vi "ziExample-Module-AWG.vi"() -> ()   [LabVIEW 2009]
doc: "Control a Zurich instrument device via the LabOne Labview API. \nRequirements: Zurich Instruments UHFLI \nThis example shows how to start a AWG module and measure it with the scope module.\n\n© Zurich Instruments AG, www.zhinst.com"
uses:
  <instrlib>/Zurich Instruments LabOne/Public/Modules/ziTypeModEnum.ctl
  <instrlib>/Zurich Instruments LabOne/Public/Configure/ziSetValueDouble.vi
  <instrlib>/Zurich Instruments LabOne/Public/Configure/ziSetValueDoubleArray.vi
  <instrlib>/Zurich Instruments LabOne/Public/Modules/ziModSetValueBinary.vi
  <instrlib>/Zurich Instruments LabOne/Public/Modules/ziModSetValueDoubleArray.vi
  <instrlib>/Zurich Instruments LabOne/Public/Modules/ziModGetScopeWave.vi
  <instrlib>/Zurich Instruments LabOne/Zurich Instruments LabOne.lvlib
panel:
  out "Status":bool
  out "Finish":bool
  out "Scopeready":bool caption="scopeready"
  out "?":cluster{dbl[], "Data Float":sgl[]}[](graph)
  in  "AWG":string="// Define an integer constant\nconst N = 4096;\n// Create  Gaussian pulses with length N points,\n// amplitude +1.0, center at N/2, and a width of N/8\nwave gauss = 1.0*gauss(N, N/2, N/8);\n\nplayWave(gauss);\nsetTrigger(1);\nsetTrigger(0);"
  out "Error Out":errorcluster
  in  "Address":string="DEV"
  out "Selected Device":string
  # "ziExample-SweepModul.vi\nRequirements: UHFLI\nsee block diagram for VI description"
  # "Tested Devices:\n- UHFLI"
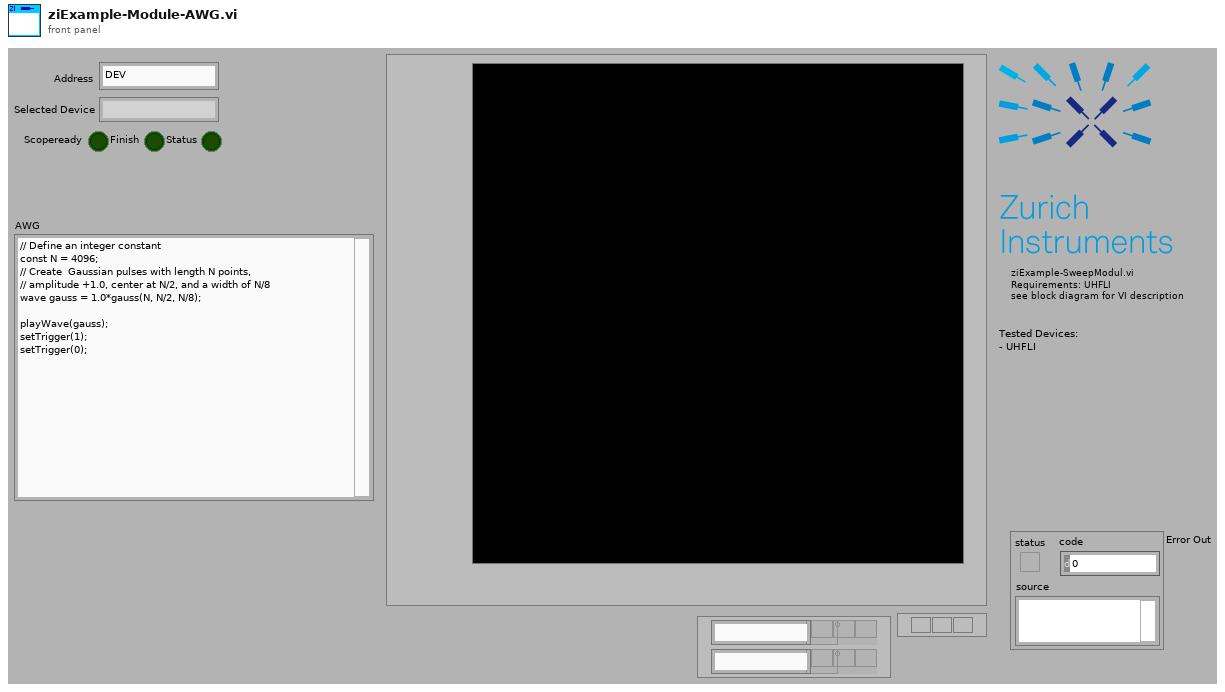
[diagram p1: front panel]
types:
  T1 = typedef "Zurich Instruments LabOne.lvlib/ziTypeModEnum.ctl" = u16
  T2 = typedef "Zurich Instruments LabOne.lvlib/ziTypeHandle.ctl" = cluster{"handleValid":bool, "Conn":u64, "Path Prefix":string, "Handle":u64, "Connected":bool, "Clockbase(s)":dbl}
  T3 = typedef "Zurich Instruments LabOne.lvlib/ziTypeModHandle.ctl" = cluster{"handleValid":bool, "Conn":u64, "ModHandle":u64, "moduleID":string, "Path Prefix":string}
  T4 = typedef "Zurich Instruments LabOne.lvlib/ziTypeModResults.ctl" = cluster{"PathArray":string[], "ValueType":T5, "NoOfResults":u64, "ziGenericHeader":T6[]}
  T5 = typedef "Zurich Instruments LabOne.lvlib/ziTypePollType.ctl" = enum16{"NONE", "DOUBLE_DATA", "INTEGER_DATA", "DEMOD_SAMPLE", "SCOPE_WAVE_HF2", "AUXIN_SAMPLE", "DIO_SAMPLE", "BYTE_ARRAY", "PWA_WAVE", "9", "10", "11", "12", "13", "14", "15", "TREE_CHANGE_DEPRI", "17", "ERROR", "19", "20", "21", "22", "23", "24", "25", "26", "27", "28", "29", "30", "31", "DOUBLE_DATA_TS", "INTEGER_DATA_TS", "34", "SCOPE_WAVE", "SCOPE_WAVE_EX", "37", "BYTE_ARRAY_TS", "39", "40", "41", "42", "43", "44", "45", "CNT_DATA", "47", "TREE_CHANGE", "49", "50", "51", "52", "53", "54", "55", "56", "57", "58", "59", "60", "61", "62", "63", "SWEEPER_DATA", "SPECTRUM_DATA", "ADVISOR_DATA", "VECTOR_DATA", "IMP_DATA"}
  T6 = typedef "Zurich Instruments LabOne.lvlib/ziTypeModGenericHeader.ctl" = cluster{"HeaderType":enum8{"HEADER_TYPE_NONE", "HEADER_TYPE_SWTRIGGER", "HEADER_TYPE_SWEEPER"}, "SampleFormat":u8, "SystemTime":timestamp, "CreatedTimeStamp":u64, "ChangedTimeStamp":u64, "Flags":u32, "ChunkSizeBytes":u64, "Name":string, "Status":u32, "GroupIndex":u32, "Color":u32, "ActiveRow":u32, "TriggerNumber":u64, "GridRows":u32, "GridCols":u32, "GridMode":u32, "GridOperation":u32, "GridDirection":u32, "GridRepetitions":u32, "GridColDelta":dbl, "GridColOffset":dbl, "GridRowDelta":dbl, "GridRowOffset":dbl, "Bandwidth":dbl, "Center":dbl, "Nenbw":dbl}
  T7 = typedef "Zurich Instruments LabOne.lvlib/ziTypeScopeWave.ctl" = cluster{"Timestamp (ticks)":u64, "Timestamp Trigger (ticks)":u64, "dt (s)":dbl, "Channel Enable":u8[], "Channel Input":enum8{"Signal Input 1", "Signal Input 2", "Trigger Input 1", "Trigger Input 2", "Aux Output 1", "Aux Output 2", "Aux Output 3", "Aux Output 4", "Aux Input 1", "Aux Input 2"}[], "Trigger Enable":u64, "Trigger Input":u64, "Channel BW Limit":u8[], "Channel Math":u8[], "Channel Scaling":sgl[], "Sequence Number":u32, "Segment Number":u32, "Block Number":u32, "Data Transfer Mode":enum8{"Single Transfer", "Block Transfer", "Continuous Transfer", "FFT Single Transfer"}, "Block Marker":enum8{"None", "End of Block"}, "Flags":u8, "Sample Format":enum8{"Int16", "Int32", "Float32", "reserved", "Int16 Interleaved", "Int32 Interleaved", "Float32 Interleaved"}, "Sample Count":u32, "Channel Offset":dbl[], "Data Int16":i16[], "Data Int32":i32[], "Data Float":sgl[], "Total Samples":u64}
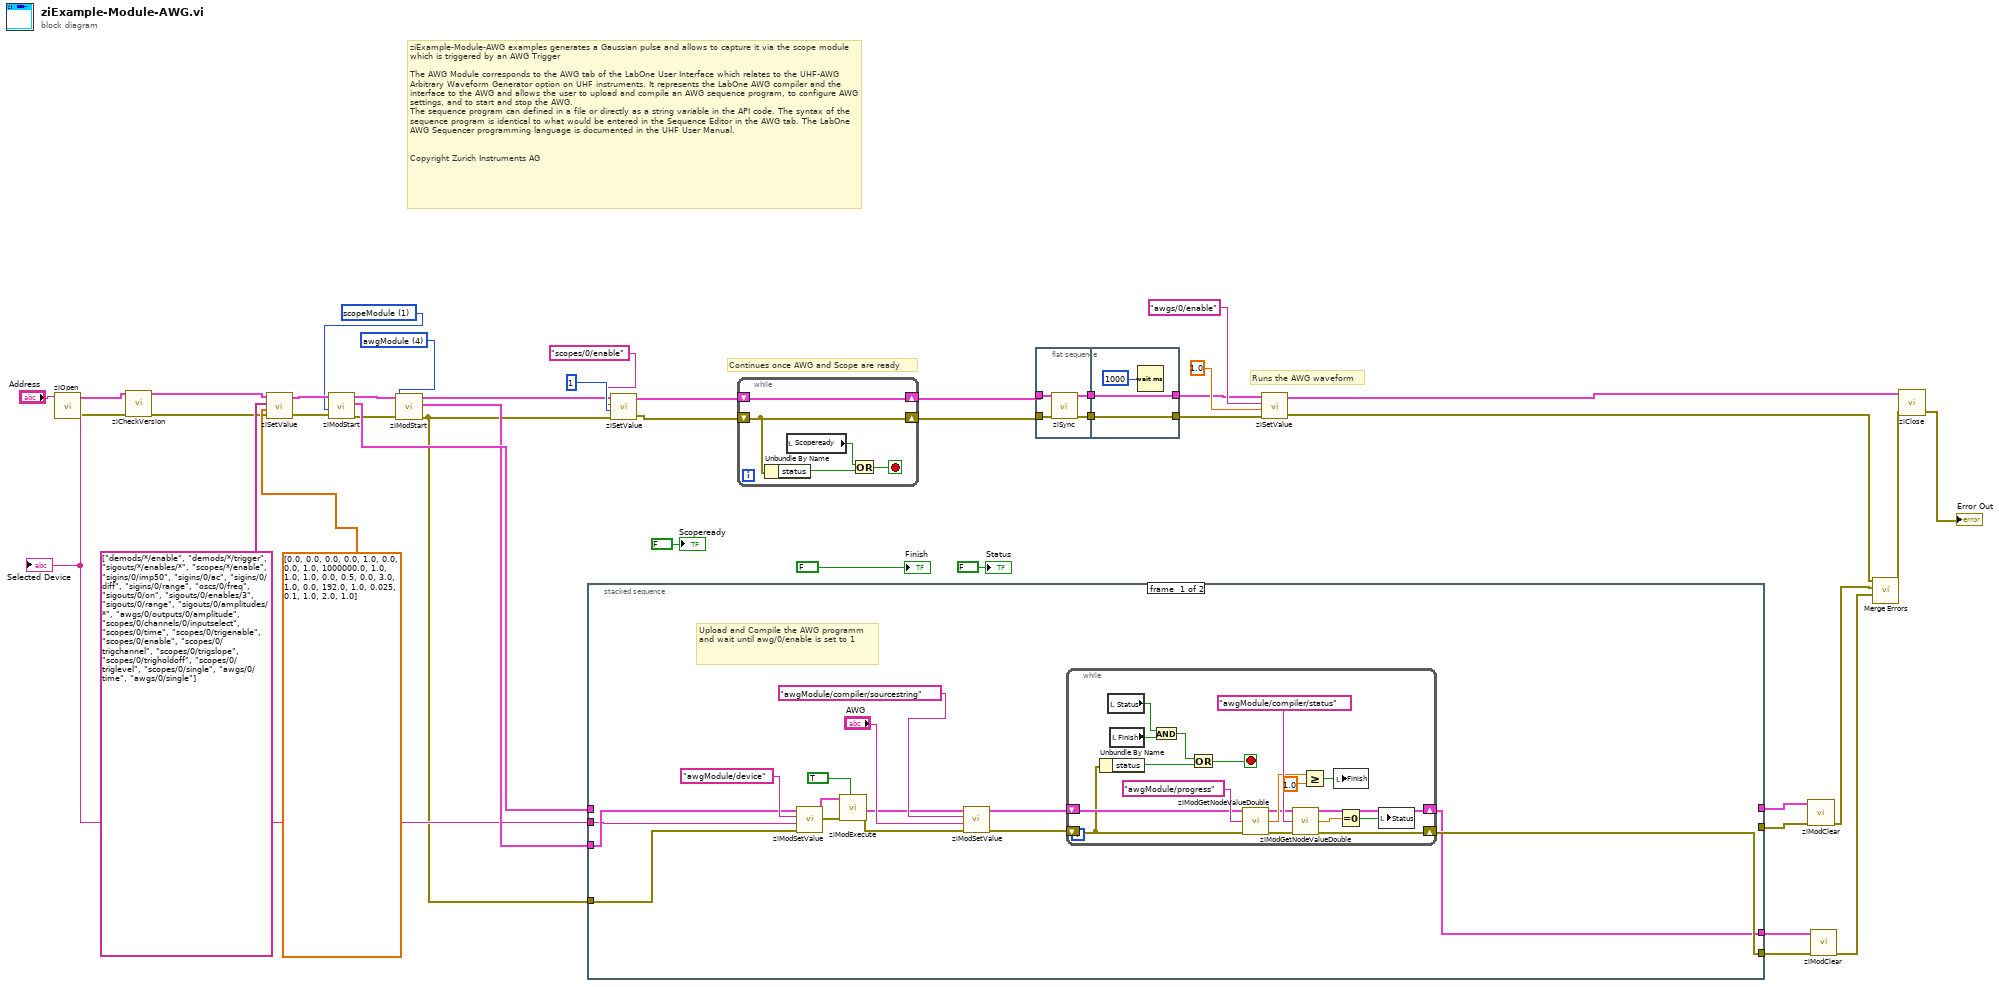
[diagram p0: block diagram]
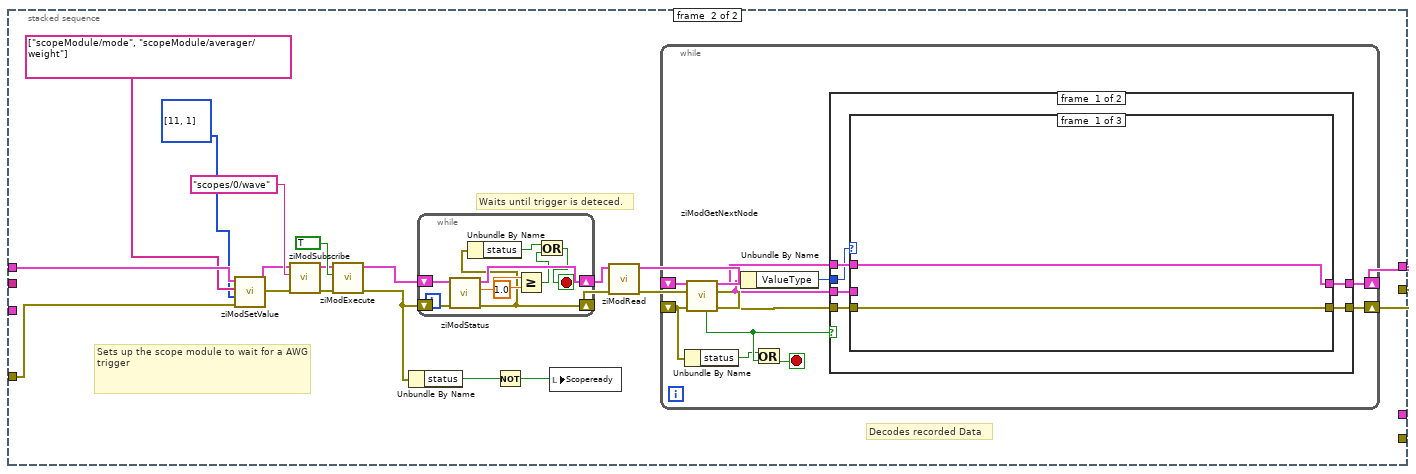
[diagram p2: hidden frame]
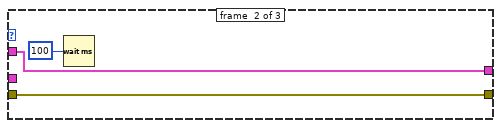
[diagram p3: hidden frame]
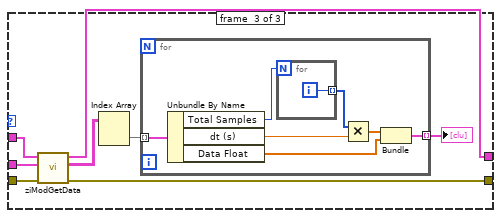
[diagram p4: hidden frame]
diagram:
  w6 = T1 4 items=["sweep", "scopeModule", "dataAcquisitionModule", "pidAdvisor", "awgModule", "impedanceModule", "multiDeviceSyncModule", "zoomFFT", "trigger", "deviceSettings", "record"] ("module Id")
  w5 = T1 1 items=["sweep", "scopeModule", "dataAcquisitionModule", "pidAdvisor", "awgModule", "impedanceModule", "multiDeviceSyncModule", "zoomFFT", "trigger", "deviceSettings", "record"] ("module Id")
  # "Runs the AWG waveform"
  # "Continues once AWG and Scope are ready"
  # "ziExample-Module-AWG examples generates a Gaussian pulse and allows to capture it via the scope module which is triggered by an AWG Trigger\n\nThe AWG Module corresponds to the AWG tab of the LabOne User Interface which relates to the UHF-AWG Arbitrary Waveform Generator option on UHF instruments. It represents the LabOne AWG compiler and the interface to the AWG and allows the user to upload and compile an AWG sequence program, to configure AWG settings, and to start and stop the AWG.\nThe sequence program can defined in a file or directly as a string variable in the API code. The syntax of the sequence program is identical to what would be entered in the Sequence Editor in the AWG tab. The LabOne AWG Sequencer programming language is documented in the UHF User Manual.\n\n\nCopyright Zurich Instruments AG"
  n1 = call <instrlib>:"ziOpen.vi"("Address"="Address") -> ("Error Out"=w10:errorcluster, "Selected Device"=w27:string, "HandleOut"=w7:T2)  [unwired: 1 in, 2 out]
  "Selected Device" <- w27
  n2 = call <instrlib>:"ziCheckVersion.vi"("Handle In"=w7, "Error In"=w10) -> ("Handle Out"=w8:T2, "Error Out"=w9:errorcluster)  [unwired: 11 in, 1 out]
  n3 = call-poly <instrlib>:"ziSetValue.vi"("Error In"=w9, "Values"=dbl[] [0.0, 0.0, 0.0, 0.0, 1.0, 0.0, 0.0, 1.0, 1000000.0, 1.0, 1.0, 1.0, 0.0, 0.5, 0.0, 3.0, 1.0, 0.0, 192.0, 1.0, 0.025, 0.1, 1.0, 2.0, 1.0], "Paths"=string[] ["demods/*/enable", "demods/*/trigger", "sigouts/*/enables/*", "scopes/*/enable", "sigins/0/imp50", "sigins/0/ac", "sigins/0/diff", "sigins/0/range", "oscs/0/freq", "sigouts/0/on", "sigouts/0/enables/3", "sigouts/0/range", "sigouts/0/amplitudes/*", "awgs/0/outputs/0/amplitude", "scopes/0/channels/0/inputselect", "scopes/0/time", "scopes/0/trigenable", "scopes/0/enable", "scopes/0/trigchannel", "scopes/0/trigslope", "scopes/0/trigholdoff", "scopes/0/triglevel", "scopes/0/single", "awgs/0/time", "awgs/0/single"], "Handle In"=w8) -> ("Error Out"=w29:errorcluster, "Handle Out"=w33:T2)  [unwired: 1 in]
  n4 = call <instrlib>:"ziModStart.vi"("Error In"=w29, "module Id"=w5, "Handle In"=w33) -> ("Error Out"=w28:errorcluster, "ModHandle Out"=w31:T3, "Handle Out"=w32:T2)  [unwired: 6 in]
  n5 = call <instrlib>:"ziModStart.vi"("Error In"=w28, "module Id"=w6, "Handle In"=w32) -> ("Error Out"=w12:errorcluster, "ModHandle Out"=w30:T3, "Handle Out"=w11:T2)  [unwired: 6 in]
  n6 = stacked-sequence {
    tunnel: w31 -> [_ w83]
    tunnel: [w54 _] -> w35
    tunnel: [w53 _] -> w36
    tunnel: [_ w85] -> w34
    tunnel: [_ w84] -> w37
    tunnel: w30 -> [w52 _]
    tunnel: w12 -> [w51 w82]
    tunnel: w27 -> [w50 _]
    frame #0 {
      # "Upload and Compile the AWG programm and wait until awg/0/enable is set to 1"
      n7 = call-poly <instrlib>:"ziModSetValue.vi"("Error In"=w51, "Data"=w50, "Path"="awgModule/device", "ModHandle In"=w52) -> ("Error Out"=w58:errorcluster, "ModHandle Out"=w57:T3)  [unwired: 6 in]
      n8 = call <instrlib>:"ziModExecute.vi"("Error In"=w58, "Modal (F)"=TRUE, "ziModHandle In"=w57) -> ("Error Out"=w46:errorcluster, "ziModHandle Out"=w47:T3)  [unwired: 5 in, 1 out]
      n9 = call-poly <instrlib>:"ziModSetValue.vi"("Error In"=w46, "Data"="AWG", "Path"="awgModule/compiler/sourcestring", "ModHandle In"=w47) -> ("Error Out"=w44:errorcluster, "ModHandle Out"=w45:T3)  [unwired: 6 in]
      n10 = while {
        shift-right: [w69] -> w53
        shift-left: w45 -> [w71]
        shift-right: [w68] -> w54
        shift-left: w44 -> [w60]
        stop <- w62 stop-if-true
        n11 = Unbundle By Name(w60) -> ("status"=w59:bool)
        n12 = local read "Status"() -> (w65:bool)
        n13 = local read "Finish"() -> (w66:bool)
        n14 = And(x=w65, y=w66) -> (x .and. y?=w61:bool)
        n15 = Or(x=w61, y=w59) -> (x .or. y?=w62:bool)
        n16 = call <instrlib>:"ziModGetNodeValueDouble.vi"("ModHandle In"=w71, "Path"="awgModule/progress", "error in"=w60) -> ("ModHandle Out"=w70:T3, "Value"=w73:dbl, "error out"=w67:errorcluster)  [unwired: 10 in]
        n17 = call <instrlib>:"ziModGetNodeValueDouble.vi"("ModHandle In"=w70, "Path"="awgModule/compiler/status", "error in"=w67) -> ("ModHandle Out"=w69:T3, "Value"=w72:dbl, "error out"=w68:errorcluster)  [unwired: 10 in]
        n18 = Greater Or Equal?(x=w73, y=1.0) -> (x >= y?=w64:bool)
        n19 = local write "Finish"(w64) -> ()
        n20 = Equal To 0?(x=w72) -> (x = 0?=w63:bool)
        n21 = local write "Status"(w63) -> ()
      }
    }
    frame #1 {
      # "Decodes recorded Data"
      # "Waits until trigger is deteced."
      # "Sets up the scope module to wait for a AWG trigger"
      n22 = call-poly <instrlib>:"ziModSetValue.vi"("Error In"=w82, "Values"=i32[] [11, 1], "Paths"=string[] ["scopeModule/mode", "scopeModule/averager/weight"], "ModHandle In"=w83) -> ("Error Out"=w89:errorcluster, "ModHandle Out"=w90:T3)  [unwired: 6 in]
      n23 = call <instrlib>:"ziModSubscribe.vi"("Error In"=w89, "Path"="scopes/0/wave", "ModHandle In"=w90) -> ("Error Out"=w87:errorcluster, "ModHandle Out"=w88:T3)  [unwired: 6 in]
      n24 = call <instrlib>:"ziModExecute.vi"("Error In"=w87, "Modal (F)"=TRUE ("Modal"), "ziModHandle In"=w88) -> ("Error Out"=w81:errorcluster, "ziModHandle Out"=w86:T3)  [unwired: 5 in, 1 out]
      n25 = Unbundle By Name(w81) -> ("status"=w80:bool)
      n26 = while {
        shift-right: [w101] -> w94
        shift-left: w86 -> [w105]
        shift-right: [w97] -> w93
        shift-left: w81 -> [w104]
        stop <- w98 stop-if-true
        n27 = call <instrlib>:"ziModStatus.vi"("Error In"=w104, "ModHandle IN"=w105) -> ("Error Out"=w97:errorcluster, "Progress (unity)"=w103:dbl, "ModHandle Out"=w101:T3)  [unwired: 5 in, 1 out]
        n28 = Unbundle By Name(w97) -> ("status"=w100:bool)
        n29 = Greater Or Equal?(x=w103, y=1.0) -> (x >= y?=w99:bool)
        n30 = Or(x=w100, y=w99) -> (x .or. y?=w98:bool)
      }
      n31 = Not(x=w80) -> (.not. x?=w77:bool)
      n32 = local write "Scopeready"(w77) -> ()
      n33 = call <instrlib>:"ziModRead.vi"("error in"=w93, "ziModHandle In"=w94) -> ("error out"=w96:errorcluster, "ziModHandle Out"=w95:T3)  [unwired: 8 in]
      n34 = while {
        shift-right: [w115] -> w84
        shift-left: w95 -> [w110]
        shift-right: [w114] -> w85
        shift-left: w96 -> [w106]
        stop <- w109 stop-if-true
        n35 = Unbundle By Name(w106) -> ("status"=w107:bool)
        n36 = call <instrlib>:"ziModGetNextNode.vi"("Error In"=w106, "ModHandle In"=w110) -> ("Error Out"=w113:errorcluster, "ModResults"=w111:T4, "ModHandle Out"=w116:T3, "NoData"=w108:bool)  [unwired: 6 in]
        n37 = Unbundle By Name(w111) -> ("ValueType"=w112:T5)
        n38 = Or(x=w107, y=w108) -> (x .or. y?=w109:bool)
        n39 = case shown="False" w108 {
          tunnel: w116 -> [w122 w144]
          tunnel: [w121 w144] -> w115
          tunnel: [w120 w145] -> w114
          tunnel: w113 -> [w119 w145]
          tunnel: w111 -> [w118 _]
          tunnel: w112 -> [w117 _]
          frame #0 {
            n40 = case shown="\"SCOPE_WAVE_EX\"" w117 {
              tunnel: w122 -> [w124 w127 w132]
              tunnel: w118 -> [_ _ w135]
              tunnel: w119 -> [w123 w126 w134]
              tunnel: [w123 w126 w133] -> w120
              tunnel: [w124 w127 w131] -> w121
              frame #0 {
              }
              frame #1 {
                n41 = Wait (ms)(milliseconds to wait=u32 100) -> ()  [unwired: 1 out]
              }
              frame #2 {
                n42 = call-poly <instrlib>:"ziModGetData.vi"("Error In"=w134, "ModResults"=w135, "ModHandle In"=w132) -> ("Error Out"=w133:errorcluster, "ModScopeWave"=w129:T7[][], "ModHandle Out"=w131:T3)  [unwired: 5 in, 1 out]
                n43 = Index Array(array=w129) -> (element=w128:T7[])  [unwired: 2 in]
                n44 = for {
                  tunnel: w128 -> [w142] mode=indexing
                  tunnel: [w141] -> w130 mode=indexing
                  n45 = Unbundle By Name(w142) -> ("Total Samples"=w138:u64, "dt (s)"=w139:dbl, "Data Float"=w140:sgl[])
                  n46 = for {
                    N: w138 -> [_]
                    tunnel: [w143] -> w136 mode=indexing
                    i -> [w143]
                  }
                  n47 = Multiply(x=w136, y=w139) -> (x*y=w137:dbl[])
                  n48 = Bundle(w137, "Data Float"=w140) -> (w141:cluster{dbl[], "Data Float":sgl[]})  [unwired: 1 in]
                }
                "?" <- w130
              }
            }
          }
          frame #1 {
          }
        }
      }
    }
  }
  n49 = call-poly <instrlib>:"ziSetValue.vi"("Error In"=w12, "Value"=1, "Path"="scopes/0/enable", "Handle In"=w11) -> ("Error Out"=w13:errorcluster, "Handle Out"=w14:T2)  [unwired: 1 in]
  n50 = while {
    shift-right: [w149] -> w3
    shift-left: w13 -> [w149]
    shift-right: [w150] -> w4
    shift-left: w14 -> [w150]
    stop <- w146 stop-if-true
    n51 = Unbundle By Name(w149) -> ("status"=w148:bool)
    n52 = local read "Scopeready"() -> (w147:bool)
    n53 = Or(x=w147, y=w148) -> (x .or. y?=w146:bool)
  }
  n54 = flat-sequence {
    tunnel: w3 -> [w154]
    tunnel: w4 -> [w151]
    tunnel: [w153] -> w2
    tunnel: [w152] -> w1
    tunnel: [w156] -> w21
    tunnel: [w157] -> w22
    tunnel: w2 -> [w157]
    tunnel: w1 -> [w156]
    frame #0 {
      n55 = call <instrlib>:"ziSync.vi"("Handle In"=w151, "Error In"=w154) -> ("Handle Out"=w152:T2, "Error Out"=w153:errorcluster)  [unwired: 12 in]
    }
    frame #1 {
      n56 = Wait (ms)(milliseconds to wait=u32 1000) -> ()  [unwired: 1 out]
    }
  }
  n57 = call-poly <instrlib>:"ziSetValue.vi"("Error In"=w22, "Value"=1.0, "Path"="awgs/0/enable", "Handle In"=w21) -> ("Error Out"=w17:errorcluster, "Handle Out"=w39:T2)  [unwired: 1 in]
  n58 = call <instrlib>:"ziModClear.vi"("Error In"=w34, "ziModHandle In"=w37) -> ("Error Out"=w25:errorcluster)  [unwired: 7 in, 1 out]
  n59 = call <instrlib>:"ziModClear.vi"("Error In"=w35, "ziModHandle In"=w36) -> ("Error Out"=w26:errorcluster)  [unwired: 7 in, 1 out]
  n60 = call <vilib>:"Merge Errors.vi"("error in 3 (no error)"=w26, "error in 2 (no error)"=w25, "error in 1 (no error)"=w17) -> ("error out"=w38:errorcluster)  [unwired: 4 in]
  n61 = call <instrlib>:"ziClose.vi"("Error In"=w38, "Handle In"=w39) -> ("Error Out"=→"Error Out":errorcluster)  [unwired: 2 in, 1 out]
  "Finish" <- FALSE ("Finish")
  "Status" <- FALSE ("Status")
  "Scopeready" <- FALSE ("scopeready")
